vi "PDE Thermal Distribution_Dirichlet Boundary.vi"(2 "data":variant, 3 "y":dbl, 4 "x":dbl, 5 "t":dbl) -> (0 "error out":errorcluster, 1 "F(t, x, y)":dbl)   [LabVIEW 2023]
doc: "This VI implements the boundary condition."
panel:
  # "This is an example of a VI that the PDE solver can call by reference. All VIs called by the PDE solver must have the same connector pane."
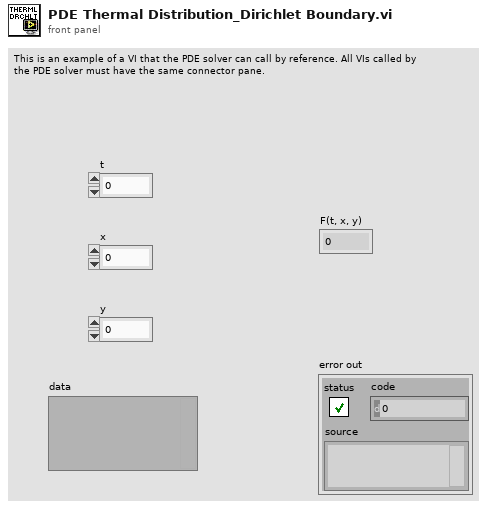
[diagram p1: front panel]
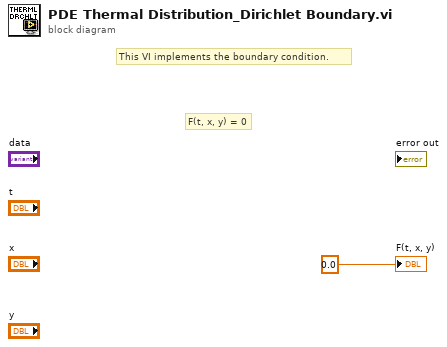
[diagram p0: block diagram]
diagram:
  # "This VI implements the boundary condition."
  # "F(t, x, y) = 0"
  "F(t, x, y)" <- 0.0 ("F(t, x, y)")
